vi "S2C_XML_CreateTest.vi"(8 "Error In":errorcluster, 11 "TestData":T1) -> (0 "Error Out":errorcluster)   [LabVIEW 2015]
uses:
  S2C_XML_Globals.vi
  <vilib>/xml/Close Reference(Node).vi
  <resource>/objmgr/DOMUserDefRef.rc
  <vilib>/xml/NI_XML.lvlib
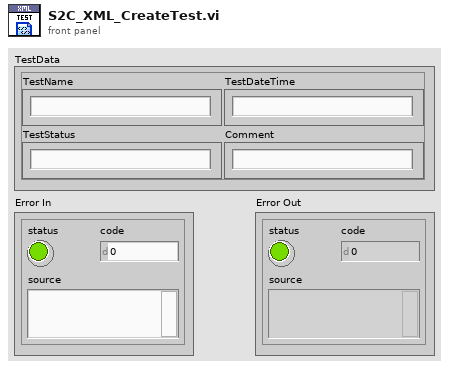
[diagram p1: front panel]
types:
  T1 = cluster{"TestName":string, "TestDateTime":string, "TestStatus":string, "Comment":string}
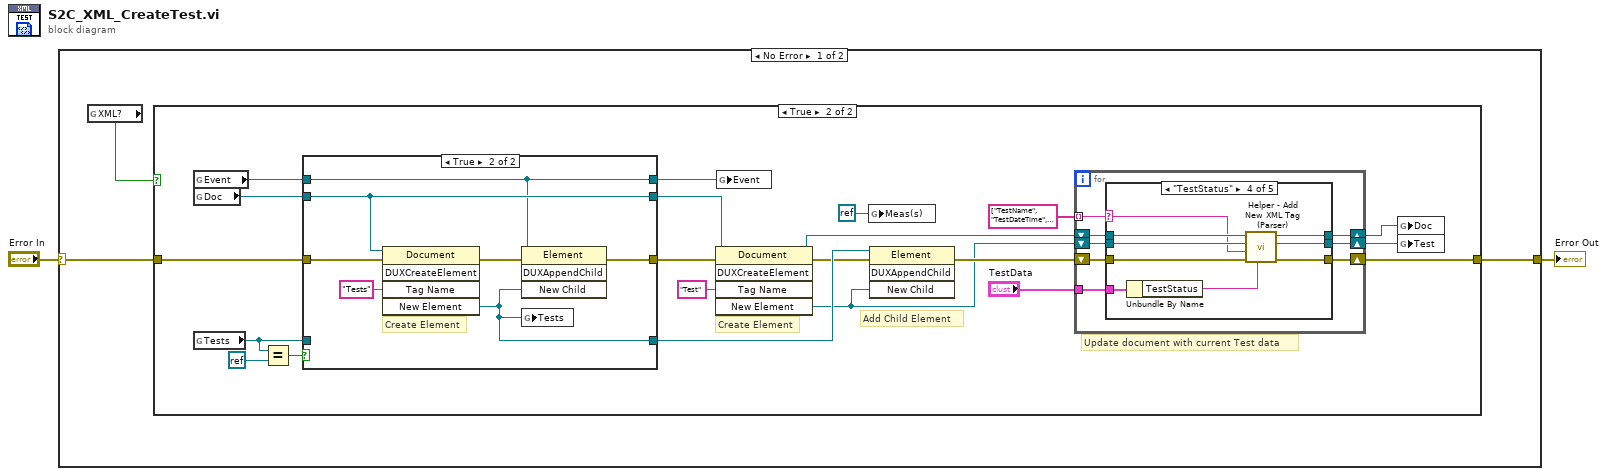
[diagram p0: block diagram]
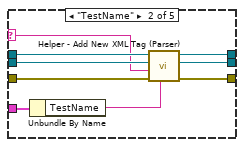
[diagram p4: hidden frame]
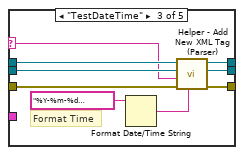
[diagram p5: hidden frame]
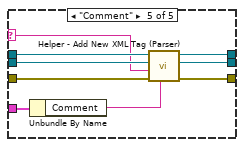
[diagram p6: hidden frame]
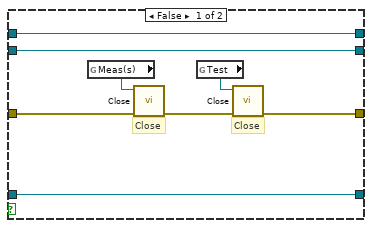
[diagram p7: hidden frame]
diagram:
  n1 = case shown="No Error" "Error In" {
    selector: "Error In" -> [w5 w90]
    tunnel: [w4 w90] -> w2
    frame No Error {
      n2 = global read "S2C_XML_Globals.vi" "XML?"() -> (w3:bool)
      n3 = case shown="True" w3 {
        tunnel: w5 -> [w6 w27]
        tunnel: [w6 w10] -> w4
        frame False {
          # "The XML Output is currently disabled"
        }
        frame True {
          # "Update document with current Test data"
          # "Add Child Element"
          # "Create Element"
          n4 = global read "S2C_XML_Globals.vi" "Event"() -> (w24:refnum<k20>)
          n5 = global read "S2C_XML_Globals.vi" "Doc"() -> (w25:refnum<k20>)
          n6 = global read "S2C_XML_Globals.vi" "Tests"() -> (w17:refnum<k20>)
          n7 = Equal?(x=w17, y=refnum<k0> refnum) -> (x = y?=w18:bool)
          n8 = case shown="True" w18 {
            tunnel: w27 -> [w75 w88]
            tunnel: w25 -> [w81 w85]
            tunnel: w24 -> [w82 w84]
            tunnel: [w80 w83] -> w23
            tunnel: [w78 w86] -> w22
            tunnel: [w81 w85] -> w21
            tunnel: [w82 w84] -> w20
            tunnel: w17 -> [w80 _]
            frame False {
              # "Close"
              # "Close"
              n9 = global read "S2C_XML_Globals.vi" "Meas(s)"() -> (w77:refnum<k20>)
              n10 = call-poly <vilib>:"Close.vi"("error in (no error)"=w75, "node"=w77) -> ("error out"=w76:errorcluster)  [unwired: 7 in]
              n11 = global read "S2C_XML_Globals.vi" "Test"() -> (w79:refnum<k20>)
              n12 = call-poly <vilib>:"Close.vi"("error in (no error)"=w76, "node"=w79) -> ("error out"=w78:errorcluster)  [unwired: 7 in]
            }
            frame True {
              # "Create Element"
              n13 = invoke class="Document" method="DUXCreateElement"(reference=w85, error in=w88, "Tag Name"="Tests") -> (error out=w87:errorcluster, "New Element"=w83:refnum<k20>)  [unwired: 2 in, 3 out]
              n14 = invoke class="Element" method="DUXAppendChild"(reference=w84, error in=w87, "New Child"=w83) -> (error out=w86:errorcluster)  [unwired: 1 in, 3 out]
              n15 = global write "S2C_XML_Globals.vi" "Tests"(w83) -> ()
            }
          }
          n16 = invoke class="Document" method="DUXCreateElement"(reference=w21, error in=w22, "Tag Name"="Test") -> (reference out=w13:refnum<k20>, error out=w16:errorcluster, "New Element"=w14:refnum<k20>)  [unwired: 2 in, 2 out]
          n17 = global write "S2C_XML_Globals.vi" "Event"(w20) -> ()
          n18 = global write "S2C_XML_Globals.vi" "Meas(s)"(refnum<k0> refnum) -> ()
          n19 = invoke class="Element" method="DUXAppendChild"(reference=w23, error in=w16, "New Child"=w14) -> (error out=w15:errorcluster)  [unwired: 1 in, 3 out]
          n20 = for {
            tunnel: string[] ["TestName", "TestDateTime", "TestStatus", "Comment"] -> [w34] mode=indexing
            shift-right: [w28] -> w8
            shift-left: w13 -> [w33]
            shift-right: [w29] -> w9
            shift-left: w14 -> [w32]
            shift-right: [w30] -> w10
            shift-left: w15 -> [w35]
            tunnel: "TestData" -> [w31]
            n21 = case shown="\"TestStatus\"" w34 {
              selector: w34 -> [_ w40 w50 w58 w67]
              tunnel: w35 -> [w36 w46 w56 w64 w73]
              tunnel: w33 -> [w38 w43 w53 w61 w70]
              tunnel: [w38 w42 w52 w60 w69] -> w28
              tunnel: w32 -> [w37 w44 w54 w62 w71]
              tunnel: [w37 w41 w51 w59 w68] -> w29
              tunnel: [w36 w45 w55 w63 w72] -> w30
              tunnel: w31 -> [_ w47 _ w65 w74]
              frame "Unknown", Default {
              }
              frame "TestName" {
                n22 = Unbundle By Name(w47) -> ("TestName"=w39:string)
                n23 = call "Helper - Add New XML Tag (Parser).vi"("Tag Data"=w39, "error in (no error)"=w46, "Tag Name"=w40, "Owning Element"=w44, "DOM document"=w43) -> ("error out"=w45:errorcluster, "dup Owning Element"=w41:refnum<k20>, "dup DOM document"=w42:refnum<k20>)  [unwired: 4 in]
              }
              frame "TestDateTime" {
                # "Format Time"
                n24 = Format Date/Time String(time format string (%c)="%Y-%m-%d %H:%M:%S%3u") -> (date/time string=w48:string)  [unwired: 2 in]
                n25 = call "Helper - Add New XML Tag (Parser).vi"("Tag Data"=w48, "error in (no error)"=w56, "Tag Name"=w50, "Owning Element"=w54, "DOM document"=w53) -> ("error out"=w55:errorcluster, "dup Owning Element"=w51:refnum<k20>, "dup DOM document"=w52:refnum<k20>)  [unwired: 4 in]
              }
              frame "TestStatus" {
                n26 = Unbundle By Name(w65) -> ("TestStatus"=w57:string)
                n27 = call "Helper - Add New XML Tag (Parser).vi"("Tag Data"=w57, "error in (no error)"=w64, "Tag Name"=w58, "Owning Element"=w62, "DOM document"=w61) -> ("error out"=w63:errorcluster, "dup Owning Element"=w59:refnum<k20>, "dup DOM document"=w60:refnum<k20>)  [unwired: 4 in]
              }
              frame "Comment" {
                n28 = Unbundle By Name(w74) -> ("Comment"=w66:string)
                n29 = call "Helper - Add New XML Tag (Parser).vi"("Tag Data"=w66, "error in (no error)"=w73, "Tag Name"=w67, "Owning Element"=w71, "DOM document"=w70) -> ("error out"=w72:errorcluster, "dup Owning Element"=w68:refnum<k20>, "dup DOM document"=w69:refnum<k20>)  [unwired: 4 in]
              }
            }
          }
          n30 = global write "S2C_XML_Globals.vi" "Doc"(w8) -> ()
          n31 = global write "S2C_XML_Globals.vi" "Test"(w9) -> ()
        }
      }
    }
    frame Error {
    }
  }
  "Error Out" <- w2
